vi "N58_coordinators.vi"(3 "DUT":i32=2) -> (0 "Message Array":string[](array[string]), 1 "String":string)   [LabVIEW 2024]
uses:
  Launcher/SubVI/Global 1.vi
  Launcher/Launcher_DTU.lvlib
panel:
  in  "N582":bool
  in  "N581":bool
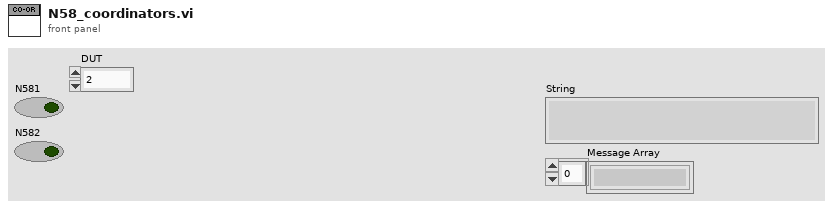
[diagram p1: front panel]
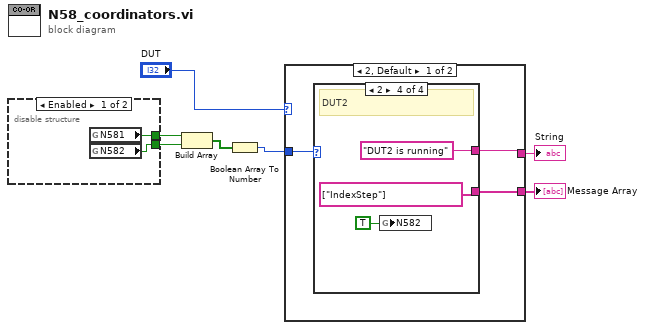
[diagram p0: block diagram]
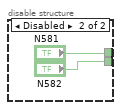
[diagram p2: hidden frame]
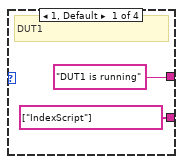
[diagram p3: hidden frame]
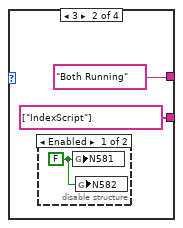
[diagram p4: hidden frame]
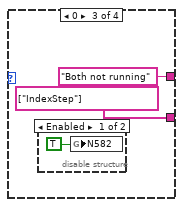
[diagram p6: hidden frame]
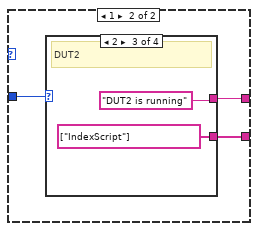
[diagram p8: hidden frame]
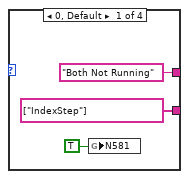
[diagram p9: hidden frame]
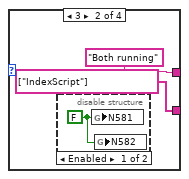
[diagram p10: hidden frame]
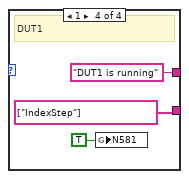
[diagram p12: hidden frame]
diagram:
  n1 = disable-structure shown="Enabled" {
    disable-tunnel: [w9 "N581"] -> w7
    disable-tunnel: [w8 "N582"] -> w6
    frame Enabled {
      n2 = global read "Global 1.vi" "N581"() -> (w9:bool)
      n3 = global read "Global 1.vi" "N582"() -> (w8:bool)
    }
    frame Disabled {
    }
  }
  n4 = Build Array(w7, w6) -> (w2:bool[])
  n5 = Boolean Array To Number(Boolean array=w2) -> (number=w1:u32)
  n6 = case shown="2, Default" "DUT" {
    tunnel: w1 -> [w14 w28]
    tunnel: [w13 w27] -> w4
    tunnel: [w12 w26] -> w3
    frame 2, Default {
      n7 = case shown="2" w14 {
        tunnel: ["DUT1 is running" "Both Running" "Both not running" "DUT2 is running"] -> w13
        tunnel: [string[] ["IndexScript"] ("Message Array") string[] ["IndexScript"] ("Message Array") string[] ["IndexStep"] ("Message Array") string[] ["IndexStep"] ("Message Array")] -> w12
        frame 1, Default {
          # "DUT1"
        }
        frame 3 {
          n8 = disable-structure shown="Enabled" {
            frame Enabled {
              w19 = FALSE ("N581")
              n9 = global write "Global 1.vi" "N581"(w19) -> ()
              n10 = global write "Global 1.vi" "N582"(w19) -> ()
            }
            frame Disabled {
            }
          }
        }
        frame 0 {
          n11 = disable-structure shown="Enabled" {
            frame Enabled {
              n12 = global write "Global 1.vi" "N582"(TRUE ("N582")) -> ()
            }
            frame Disabled {
            }
          }
        }
        frame 2 {
          # "DUT2"
          n13 = global write "Global 1.vi" "N582"(TRUE ("N582")) -> ()
        }
      }
    }
    frame 1 {
      n14 = case shown="2" w28 {
        tunnel: ["Both Not Running" "Both running" "DUT2 is running" "DUT1 is running"] -> w27
        tunnel: [string[] ["IndexStep"] ("Message Array") string[] ["IndexScript"] ("Message Array") string[] ["IndexScript"] ("Message Array") string[] ["IndexStep"] ("Message Array")] -> w26
        frame 0, Default {
          n15 = global write "Global 1.vi" "N581"(TRUE ("N581")) -> ()
        }
        frame 3 {
          n16 = disable-structure shown="Enabled" {
            frame Enabled {
              w34 = FALSE ("N581")
              n17 = global write "Global 1.vi" "N581"(w34) -> ()
              n18 = global write "Global 1.vi" "N582"(w34) -> ()
            }
            frame Disabled {
            }
          }
        }
        frame 2 {
          # "DUT2"
        }
        frame 1 {
          # "DUT1"
          n19 = global write "Global 1.vi" "N581"(TRUE ("N581")) -> ()
        }
      }
    }
  }
  "String" <- w4
  "Message Array" <- w3
